vi "CreateHTML.vi"(0 "reference in":refnum<class "Graph.lvclass">, 2 "VI Name":string, 5 "error in (no error)":errorcluster) -> (13 "script dependencies":string[](array[string]), 14 "reference out":refnum<class "Graph.lvclass">, 15 "HTML":string, 16 "js variables":string, 17 "js code for controls":string, 18 "js code for indicators":string, 19 "error out":errorcluster)   [LabVIEW 2014, in "Graph.lvclass"]
uses:
  Graph.lvclass
  Object_class/Object.lvclass
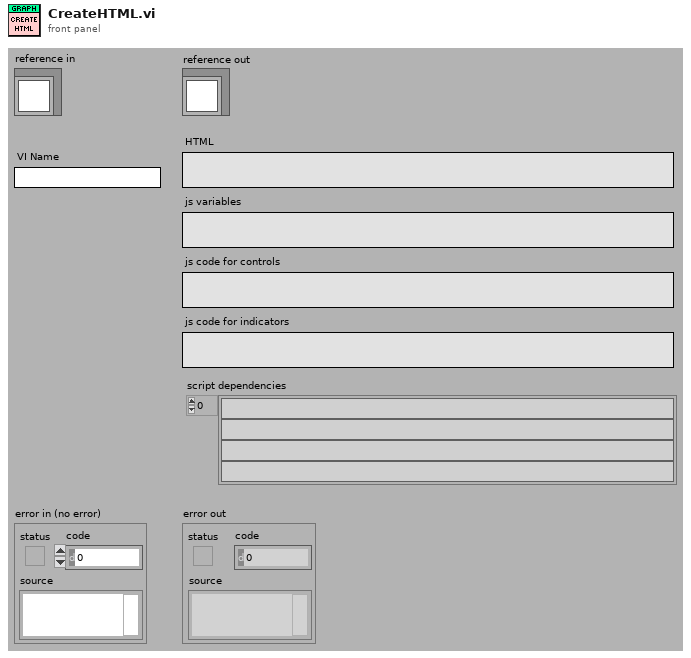
[diagram p1: front panel]
types:
  T1 = typedef "Object.lvclass/Attributes.ctl" = cluster{"UID":i32, "Type":string, "Coordinates":T2, "Reference":refnum<vi>}
  T2 = typedef "Object.lvclass/Coordinates.ctl" = cluster{"Left":i32, "Top":i32, "Height":u32, "Width":u32}
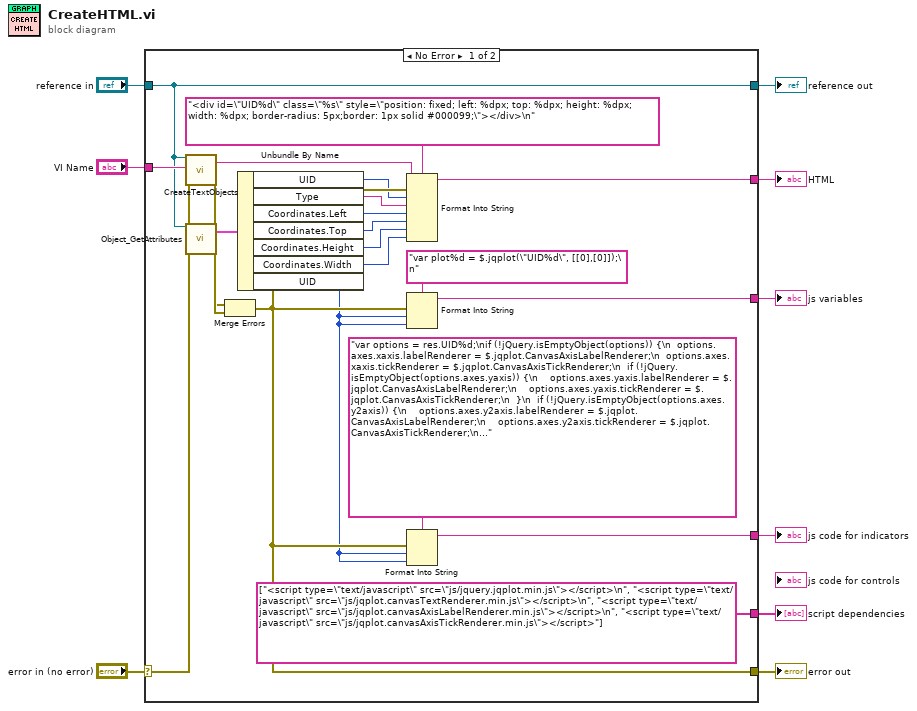
[diagram p0: block diagram]
diagram:
  n1 = case shown="No Error" "error in (no error)" {
    selector: "error in (no error)" -> [w29 w33]
    tunnel: [w28 w33] -> w8
    tunnel: [w20 _] -> w7
    tunnel: [w14 _] -> w6
    tunnel: [w13 _] -> w5
    tunnel: [string[] ["<script type=\"text/javascript\" src=\"js/jquery.jqplot.min.js\"></script>\n", "<script type=\"text/javascript\" src=\"js/jqplot.canvasTextRenderer.min.js\"></script>\n", "<script type=\"text/javascript\" src=\"js/jqplot.canvasAxisLabelRenderer.min.js\"></script>\n", "<script type=\"text/javascript\" src=\"js/jqplot.canvasAxisTickRenderer.min.js\"></script>"] _] -> w4
    tunnel: "VI Name" -> [w16 _]
    tunnel: [w11 w32] -> w2
    tunnel: "reference in" -> [w11 w32]
    frame No Error {
      n2 = call-dynamic "CreateTextObjects.vi"("reference in"=w11, "VI Name"=w16, "error in (no error)"=w29) -> ("HTML"=w17:string, "error out"=w30:errorcluster)  [unwired: 14 in, 1 out]
      n3 = call "Object_GetAttributes.vi"("reference in"=w11, "error in (no error)"=w29) -> ("Data"=w19:T1, "error out"=w31:errorcluster)  [unwired: 14 in, 2 out]
      n4 = Merge Errors(w30, w31) -> (w28:errorcluster)
      n5 = Unbundle By Name(w19) -> ("UID"=w26:i32, "Type"=w25:string, "Coordinates.Left"=w24:i32, "Coordinates.Top"=w23:i32, "Coordinates.Height"=w22:u32, "Coordinates.Width"=w21:u32, "UID"=w10:i32)
      n6 = Format Into String(format string="<div id=\"UID%d\" class=\"%s\" style=\"position: fixed; left: %dpx; top: %dpx; height: %dpx; width: %dpx; border-radius: 5px;border: 1px solid #000099;\"></div>\n", initial string=w17, error in=w28, w26, w25, w24, w23, w22, w21) -> (resulting string=w20:string)  [unwired: 1 out]
      n7 = Format Into String(format string="var plot%d = $.jqplot(\"UID%d\", [[0],[0]]);\n", error in=w28, w10, w10) -> (resulting string=w14:string)  [unwired: 1 in, 1 out]
      n8 = Format Into String(format string="var options = res.UID%d;\nif (!jQuery.isEmptyObject(options)) {\n  options.axes.xaxis.labelRenderer = $.jqplot.CanvasAxisLabelRenderer;\n  options.axes.xaxis.tickRenderer = $.jqplot.CanvasAxisTickRenderer;\n  if (!jQuery.isEmptyObject(options.axes.yaxis)) {\n    options.axes.yaxis.labelRenderer = $.jqplot.CanvasAxisLabelRenderer;\n    options.axes.yaxis.tickRenderer = $.jqplot.CanvasAxisTickRenderer;\n  }\n  if (!jQuery.isEmptyObject(options.axes.y2axis)) {\n    options.axes.y2axis.labelRenderer = $.jqplot.CanvasAxisLabelRenderer;\n    options.axes.y2axis.tickRenderer = $.jqplot.CanvasAxisTickRenderer;\n  }\n  plot%d.replot(options);\n}\n", error in=w28, w10, w10) -> (resulting string=w13:string)  [unwired: 1 in, 1 out]
    }
    frame Error {
    }
  }
  "error out" <- w8
  "reference out" <- w2
  "HTML" <- w7
  "js variables" <- w6
  "script dependencies" <- w4
  "js code for indicators" <- w5
